vi "test Deployment Switch and RaF No Routing Channels.vi"(8 "error in (no error)":errorcluster, 11 "TestCase in":refnum<class "Routing and Faulting System Tests.lvclass">) -> (0 "error out":errorcluster, 3 "TestCase out":refnum<class "Routing and Faulting System Tests.lvclass">)   [LabVIEW 2017, in "Routing and Faulting System Tests.lvclass"]
uses:
  Routing and Faulting System Tests.lvclass
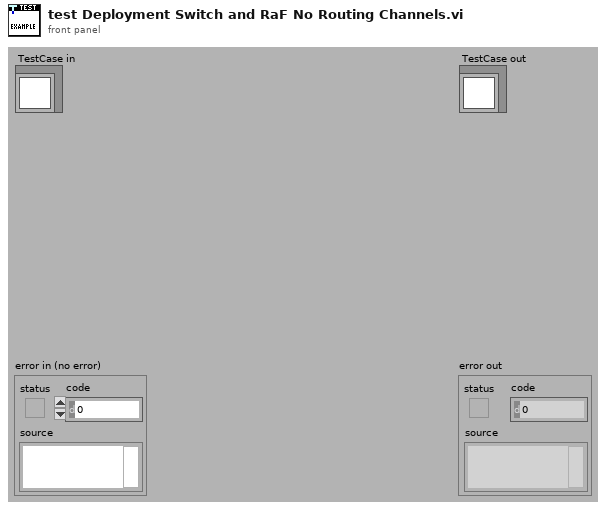
[diagram p1: front panel]
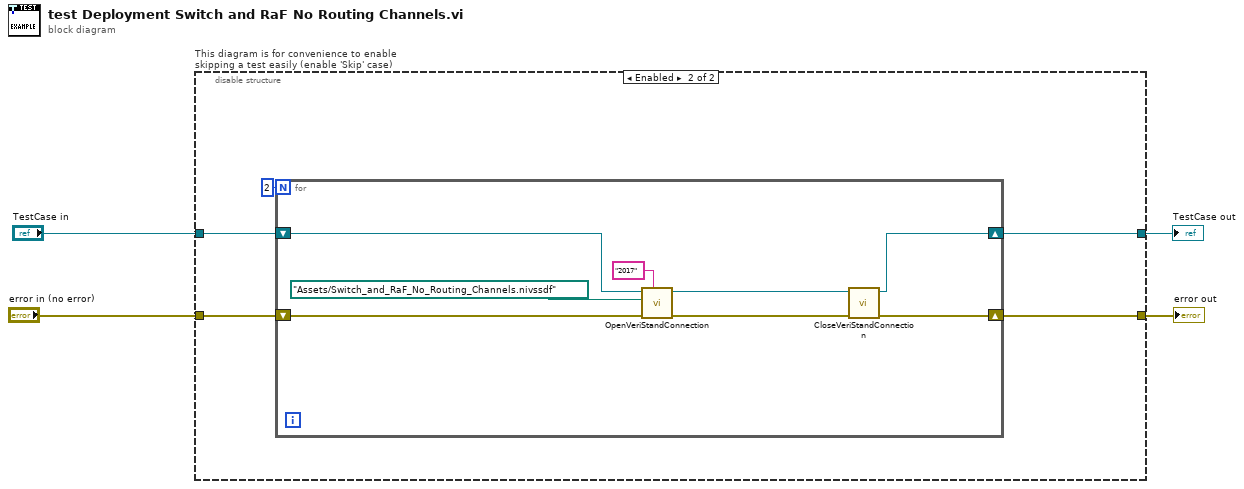
[diagram p0: block diagram]
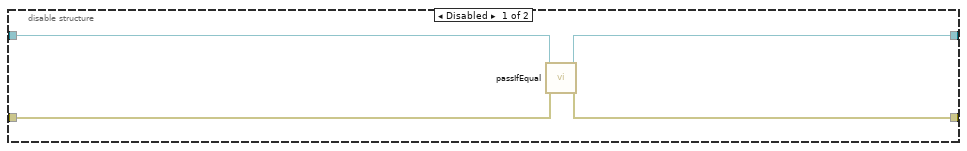
[diagram p2: hidden frame]
diagram:
  n1 = disable-structure "This diagram is for convenience to enable skipping a test easily (enable 'Skip' case)" shown="Enabled" {
    disable-tunnel: "TestCase in" -> [w8 w13]
    disable-tunnel: [w7 w10] -> w1
    disable-tunnel: [w6 w9] -> w3
    disable-tunnel: "error in (no error)" -> [w5 w12]
    frame Disabled {
      n2 = call-dynamic "passIfEqual.vi"("error in (no error)"=w5, "TestCase in"=w8) -> ("error out"=w6:errorcluster, "TestCase out"=w7:refnum<class "Routing and Faulting System Tests.lvclass">)  [unwired: 8 in]
    }
    frame Enabled {
      n3 = for {
        N: 2 -> [_]
        shift-right: [w17] -> w10
        shift-left: w13 -> [w19]
        shift-right: [w16] -> w9
        shift-left: w12 -> [w18]
        n4 = call-dynamic "OpenVeriStandConnection.vi"("Minimum VeriStand Version (2015)"="2017", "error in (no error)"=w18, "System Definition File"=path "Assets/Switch_and_RaF_No_Routing_Channels.nivssdf", "VeriStand Test Case in"=w19) -> ("error out"=w14:errorcluster, "VeriStand Test Case out"=w15:refnum<class "Routing and Faulting System Tests.lvclass">)  [unwired: 5 in, 1 out]
        n5 = call-dynamic "CloseVeriStandConnection.vi"("error in (no error)"=w14, "VeriStand Test Case in"=w15) -> ("error out"=w16:errorcluster, "VeriStand Test Case out"=w17:refnum<class "Routing and Faulting System Tests.lvclass">)  [unwired: 8 in]
      }
    }
  }
  "error out" <- w3
  "TestCase out" <- w1
